vi "Write Analog Variable Setups toIni.vi"(0 "error in (no error)":errorcluster, 2 "Path":path, 7 "Enum with Variable List":variant, 11 "Analog User settigns":T1[](array[typedef]) {"Scaling"."Offset" format="%.5f"; "Scaling"."Gain" format="%.5f"; "Limits and responces"."Limits"."H" format="%.3f"; "Limits and responces"."Limits"."L" format="%.3f"; "Limits and responces"."Limits"."HH" format="%.3f"; "Limits and responces"."Limits"."LL" format="%.3f"}, 12 "Section(\"Default\")":string="Default") -> (4 "error out":errorcluster)   [LabVIEW 2011]
uses:
  User Setting Analog Channel Bg.ctl
  Scaling.ctl
  Alarm Setup Analog.ctl
  Alarm Responce.ctl
  Action List.ctl
  Limits.ctl
  <vilib>/Utility/VariantDataType/GetNumericInfo.vi
  <vilib>/Utility/libraryn.llb/Check if File or Folder Exists.vi
  <vilib>/Utility/config.llb/NI_LVConfig.lvlib
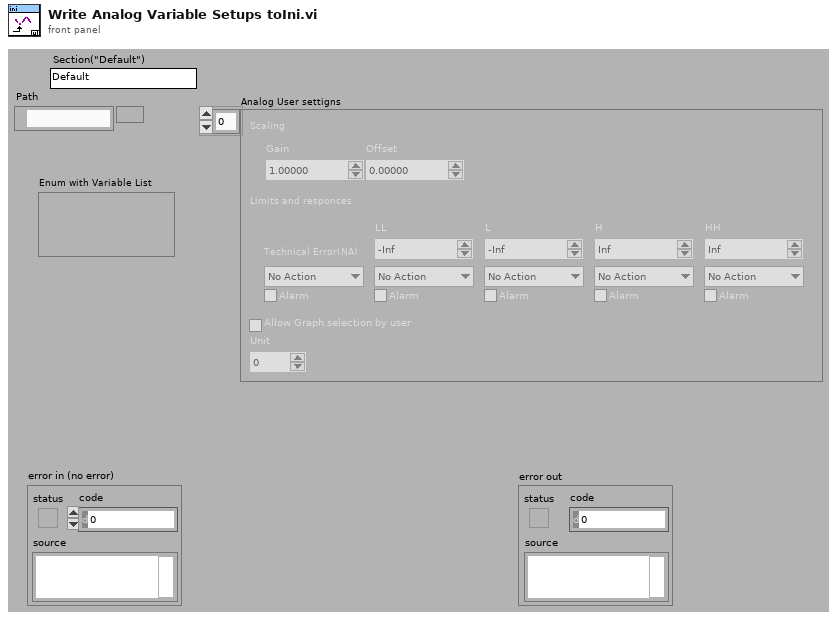
[diagram p1: front panel]
types:
  T1 = typedef "User Setting Analog Channel Bg.ctl" = cluster{"Scaling":T2, "Limits and responces":T3, "Allow Graph selection by user":bool, "Unit":u16}
  T2 = typedef "Scaling.ctl" = cluster{"Gain":dbl, "Offset":dbl}
  T3 = typedef "Alarm Setup Analog.ctl" = cluster{"Technical Error(NA)":T4, "LL":T4, "L":T4, "H":T4, "HH":T4, "Limits":T6}
  T4 = typedef "Alarm Responce.ctl" = cluster{"Action":T5, "Alarm":bool}
  T5 = typedef "Action List.ctl" = enum16{"No Action", "Stop Motor", "Turn Off HV"}
  T6 = typedef "Limits.ctl" = cluster{"LL":dbl, "L":dbl, "H":dbl, "HH":dbl}
  T7 = typedef "NI_LVConfig.lvlib/Config Data RefNum.ctl" = refnum<k1>
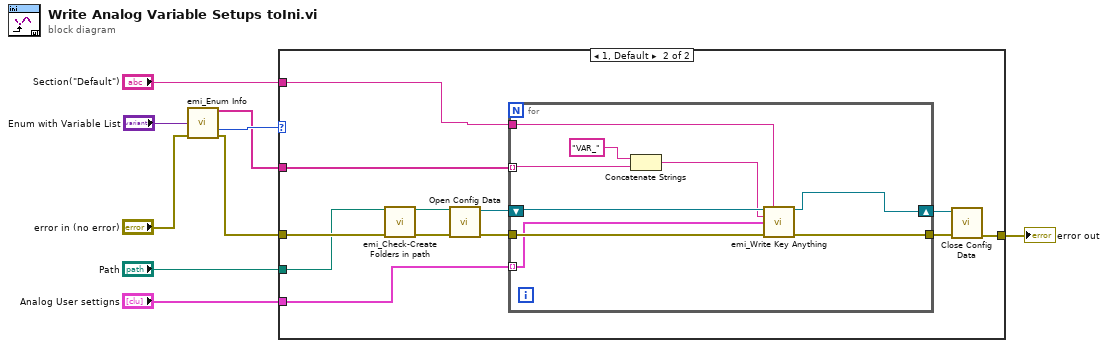
[diagram p0: block diagram]
diagram:
  n1 = call "emi_Enum Info.vi"("Enum"="Enum with Variable List", "error in (no error)"="error in (no error)") -> ("Text Elements"=w6:string[], "Numb Elements"=w7:i32, "error out"=w4:errorcluster)  [unwired: 10 in, 1 out]
  n2 = case shown="1, Default" w7 {
    tunnel: w6 -> [_ w20]
    tunnel: w4 -> [w10 w12]
    tunnel: [w10 w17] -> w9
    tunnel: "Section(\"Default\")" -> [_ w14]
    tunnel: "Analog User settigns" -> [_ w13]
    tunnel: "Path" -> [_ w11]
    frame 0 {
    }
    frame 1, Default {
      n3 = call "emi_Check-Create Folders in path.vi"("Path including file"=w11, "error in (no error)"=w12) -> ("Path out"=w15:path, "error out"=w16:errorcluster)  [unwired: 11 in, 1 out]
      n4 = call <vilib>:"Open Config Data.vi"("error in (no error)"=w16, "configuration file path"=w15) -> ("error out"=w22:errorcluster, "refnum"=w21:T7)  [unwired: 7 in, 1 out]
      n5 = for {
        tunnel: w20 -> [w25] mode=indexing
        tunnel: w22 -> [w30]
        tunnel: w14 -> [w29]
        tunnel: [w23] -> w19
        shift-right: [w26] -> w18
        shift-left: w21 -> [w28]
        tunnel: w13 -> [w24] mode=indexing
        n6 = Concatenate Strings("VAR_" ("string"), w25) -> (w27:string)
        n7 = call "emi_Write Key Anything.vi"("Ini file refnum"=w28, "Section(Default)"=w29, "Name"=w27, "Anything"=w24, "error in (no error)"=w30) -> ("Ini file refnum out"=w26:T7, "error out"=w23:errorcluster)  [unwired: 9 in]
      }
      n8 = call <vilib>:"Close Config Data.vi"("error in (no error)"=w19, "refnum"=w18) -> ("error out"=w17:errorcluster)  [unwired: 8 in, 1 out]
    }
  }
  "error out" <- w9
